vi "Get Description.vi"(8 "error in":errorcluster, 11 "Beverage in":refnum<class "Beverage.lvclass">) -> (0 "error out":errorcluster, 2 "Description":string, 3 "Beverage out":refnum<class "Beverage.lvclass">)   [LabVIEW 2020, in "Beverage.lvclass"]
doc: "Return a string <b>Description</b> of the Beverage object."
uses:
  Beverage.lvclass
  Beverage.lvclass/Beverage.ctl
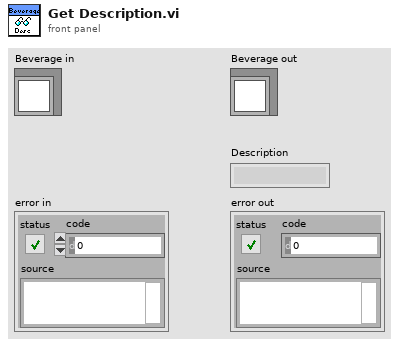
[diagram p1: front panel]
types:
  T1 = typedef "Beverage.lvclass/Drink Type.ctl" = enum16{"Dark Roast", "Decaf", "Espresso", "House Blend"}
  T2 = typedef "Beverage.lvclass/Options.ctl" = enum16{"<None>", "Milk", "Mocha", "Soy", "Whip"}
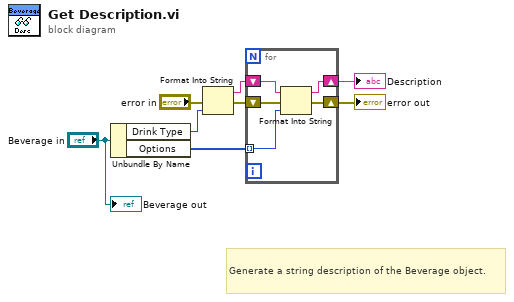
[diagram p0: block diagram]
diagram:
  # "Generate a string description of the Beverage object."
  n1 = Unbundle By Name("Beverage in") -> ("Drink Type"=w7:T1, "Options"=w6:T2[])
  n2 = Format Into String(error in="error in", w7) -> (resulting string=w5:string, error out=w3:errorcluster)  [unwired: 2 in]
  n3 = for {
    tunnel: w6 -> [w12] mode=indexing
    shift-right: [w11] -> w4
    shift-left: w5 -> [w13]
    shift-right: [w9] -> w1
    shift-left: w3 -> [w10]
    n4 = Format Into String(initial string=w13, error in=w10, w12) -> (resulting string=w11:string, error out=w9:errorcluster)  [unwired: 1 in]
  }
  "Description" <- w4
  "error out" <- w1
  "Beverage out" <- "Beverage in"
